vi "Init Module.vi"(8 "error in (no error)":errorcluster, 10 "Init Sequence":string[](array[string]), 11 "Module Refs":T1={"ModuleName"=enum."Controller", "Queue"=refnum, "user event"=refnum, "VI Refnum"=refnum, "ShowFP"=FALSE, "StatesTracking Enabled"=FALSE}) -> (0 "error out":errorcluster, 2 "queue out":refnum<queue>, 3 "Module Refs Out":T1={"ModuleName"=enum."Controller", "Queue"=refnum, "user event"=refnum, "VI Refnum"=refnum, "ShowFP"=FALSE, "StatesTracking Enabled"=FALSE}, 5 "user event out":refnum<user-event>)   [LabVIEW 2021, in "Architecture.lvlib"]
doc: "This method initializes and registers all required data for a module to be able to communicate with the others in our application. It can perform an initialization states sequence once it runs if passed throughout \"Init Sequence\" input."
uses:
  Architecture.lvlib
  Typedefs/Message.ctl
  Typedefs/Module References.ctl
  Typedefs/Enum_Module_Name.ctl
  Typedefs/FGV Ref. Modules Function.ctl
  Modules/Configuration/Configuration.lvlib
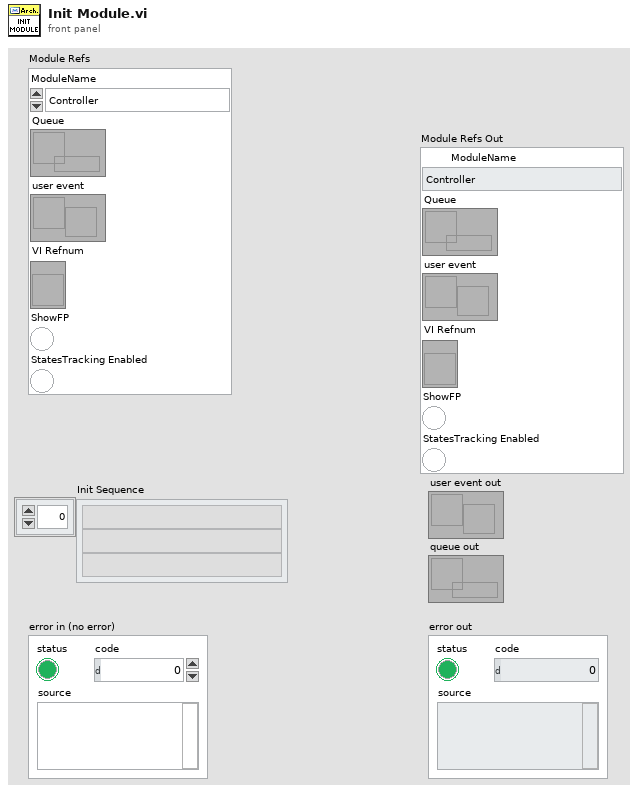
[diagram p1: front panel]
types:
  T1 = typedef "Architecture.lvlib/Module References.ctl" = cluster{"ModuleName":T2, "Queue":refnum<queue>, "user event":refnum<user-event>, "VI Refnum":refnum<vi>, "ShowFP":bool, "StatesTracking Enabled":bool}
  T2 = typedef "Configuration.lvlib/Enum_Module_Name.ctl" = enum16{"Configuration", "Error_Handler", "Log", "Database", "Controller", "UI Module"}
  T3 = typedef "Architecture.lvlib/FGV Ref. Modules Function.ctl" = enum16{"Init ", "Add Module", "Get Module", "Get All", "Add Asynchronous Run Ref", "Dispose"}
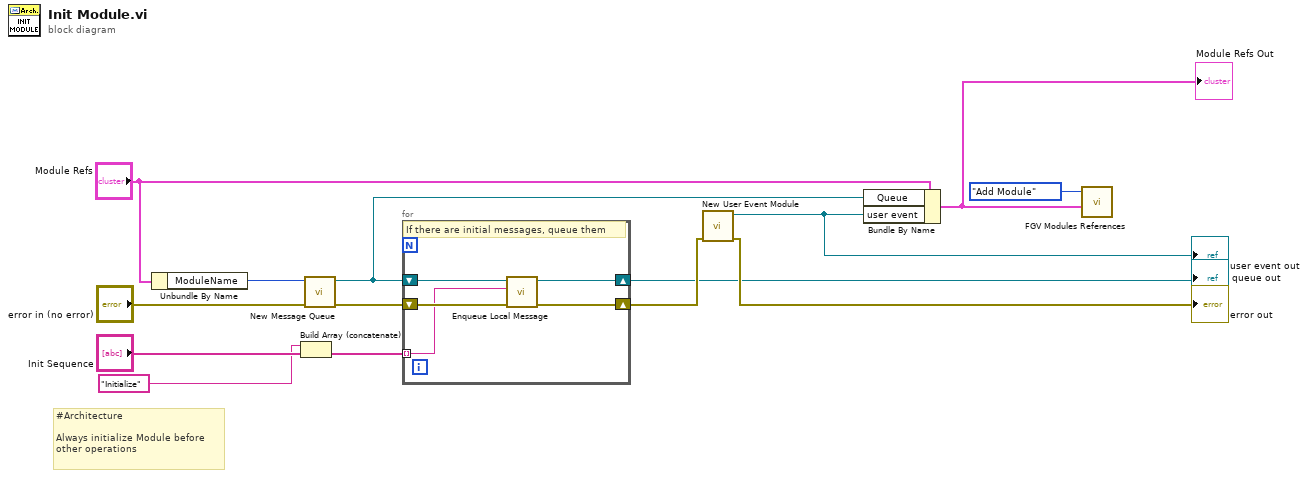
[diagram p0: block diagram]
diagram:
  # "#Architecture\n\nAlways initialize Module before \nother operations"
  n1 = Unbundle By Name("Module Refs") -> ("ModuleName"=w2:T2)
  n2 = Build Array (concatenate)("Initialize", "Init Sequence") -> (w4:string[])
  n3 = call "New Message Queue.vi"("error in (no error)"="error in (no error)", "ModuleName In"=w2) -> ("error out"=w9:errorcluster, "Msg queue out"=w7:refnum<queue>)  [unwired: 8 in]
  n4 = for {
    shift-right: [w18] -> w8
    shift-left: w9 -> [w19]
    shift-right: [w16] -> w6
    shift-left: w7 -> [w17]
    tunnel: w4 -> [w15] mode=indexing
    # "If there are initial messages, queue them"
    n5 = call "Enqueue Local Message.vi"("error in"=w19, "Message"=w15, "Msg queue in"=w17) -> ("error out"=w18:errorcluster, "queue out"=w16:refnum<queue>)  [unwired: 7 in]
  }
  "queue out" <- w6
  n6 = call "New User Event Module.vi"("error in (no error)"=w8) -> ("error out"=→"error out":errorcluster, "user event out"=w11:refnum<user-event>)  [unwired: 9 in]
  "user event out" <- w11
  n7 = Bundle By Name(cluster="Module Refs", "Queue"=w7, "user event"=w11) -> (w10:T1)
  "Module Refs Out" <- w10
  n8 = call "FGV Modules References.vi"("Module_Refs"=w10, "FGV Ref. Function In"=FGV_Ref._Modules_Function."Add Module") -> ()  [unwired: 6 in, 4 out]
